vi "FaultCheck.vi"(8 "error in (no error)":errorcluster, 10 "Cluster in":T2, 11 "Enum in":T1) -> (0 "error out":errorcluster, 2 "Cluster out":T2, 3 "Enum out":T1)   [LabVIEW 2018]
uses:
  Type_Def Actuator Controls.ctl
  Type_Def_ControlState.ctl
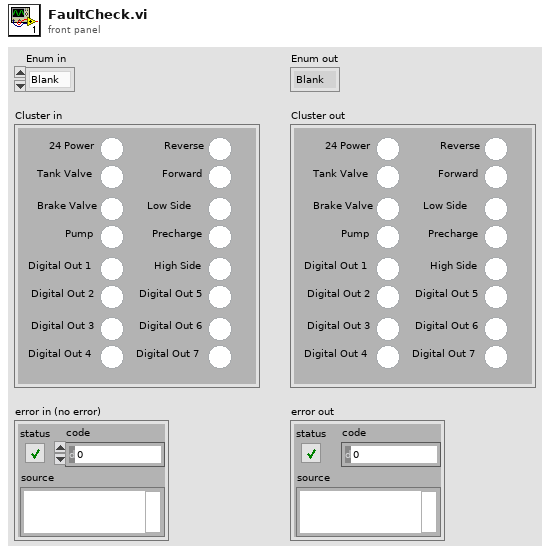
[diagram p1: front panel]
types:
  T1 = typedef "Type_Def_ControlState.ctl" = enum16{"Blank", "Systems Check", "Idle", "Ready", "Pushing", "CrawlingPrecharge", "Braking", "Fault", "Boot Up", "Unpowered", "Crawling", "Shutdown", "Service Push", "Service Wait", "Vent", "Precharge", "Cooldown"}
  T2 = typedef "Type_Def Actuator Controls.ctl" = cluster{"Reverse ":bool, "Forward":bool, "Low Side":bool, "Precharge":bool, "High Side":bool, "Digital Out 5":bool, "Digital Out 6":bool, "Digital Out 7 ":bool, "24 Power":bool, "Tank Valve ":bool, "Brake Valve":bool, "Pump":bool, "Digital Out 1 ":bool, "Digital Out 2":bool, "Digital Out 3":bool, "Digital Out 4 ":bool}
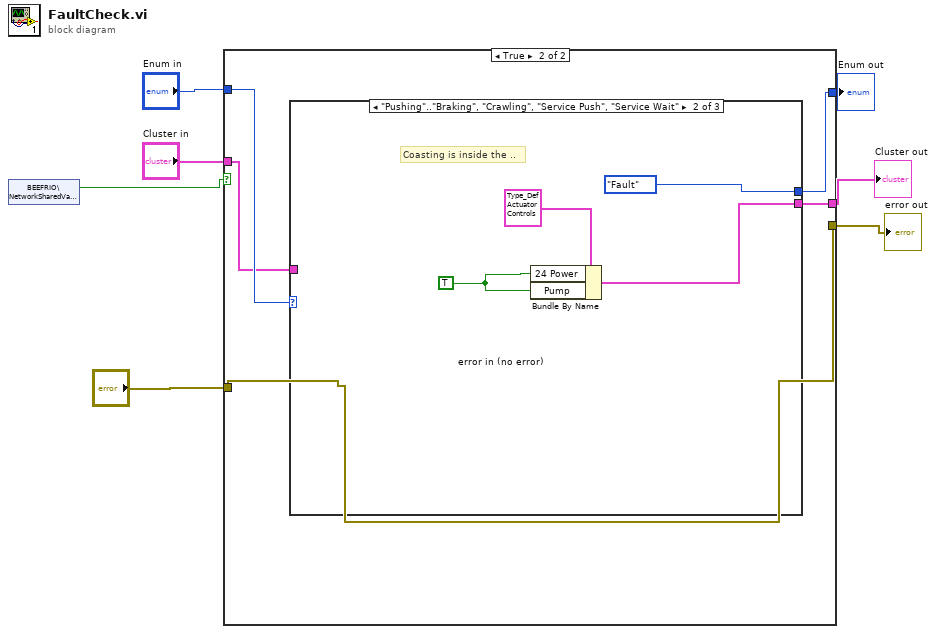
[diagram p0: block diagram]
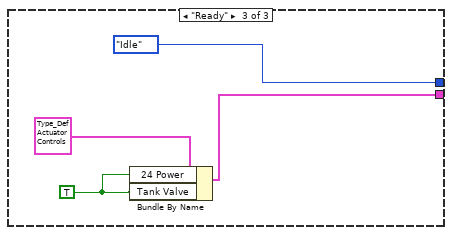
[diagram p4: hidden frame]
diagram:
  n1 = shared-variable "BEEFRIO\\NetworkSharedVariable.lvlib\\Fault"() -> (w1:bool)  [unwired: 1 in, 1 out]
  n2 = case shown="True" w1 {
    tunnel: [w10 w11] -> w7
    tunnel: "error in (no error)" -> [w10 w11]
    tunnel: [w9 w13] -> w5
    tunnel: "Cluster in" -> [w9 w12]
    tunnel: [w8 w14] -> w3
    tunnel: "Enum in" -> [w8 w15]
    frame False {
    }
    frame True {
      n3 = case shown="\"Pushing\"..\"Braking\", \"Crawling\", \"Service Push\", \"Service Wait\"" w15 {
        selector: w15 -> [w16 _ _]
        tunnel: [w16 Type_Def_ControlState."Fault" ("Enum in 2") Type_Def_ControlState."Idle" ("Enum in 2")] -> w14
        tunnel: [w17 w20 w24] -> w13
        tunnel: w12 -> [w17 _ _]
        frame Default {
        }
        frame "Pushing".."Braking", "Crawling", "Service Push", "Service Wait" {
          w18 = TRUE
          # "Coasting is inside the .."
          n4 = Bundle By Name(cluster=T2 {"Reverse "=FALSE, "Forward"=FALSE, "Low Side"=FALSE, "Precharge"=FALSE, "High Side"=FALSE, "Digital Out 5"=FALSE, "Digital Out 6"=FALSE, "Digital Out 7 "=FALSE, "24 Power"=FALSE, "Tank Valve "=FALSE, "Brake Valve"=FALSE, "Pump"=FALSE, "Digital Out 1 "=FALSE, "Digital Out 2"=FALSE, "Digital Out 3"=FALSE, "Digital Out 4 "=FALSE} ("Cluster in 2"), "24 Power"=w18, "Pump"=w18) -> (w20:T2)
        }
        frame "Ready" {
          w22 = TRUE
          n5 = Bundle By Name(cluster=T2 {"Reverse "=FALSE, "Forward"=FALSE, "Low Side"=FALSE, "Precharge"=FALSE, "High Side"=FALSE, "Digital Out 5"=FALSE, "Digital Out 6"=FALSE, "Digital Out 7 "=FALSE, "24 Power"=FALSE, "Tank Valve "=FALSE, "Brake Valve"=FALSE, "Pump"=FALSE, "Digital Out 1 "=FALSE, "Digital Out 2"=FALSE, "Digital Out 3"=FALSE, "Digital Out 4 "=FALSE} ("Cluster in 2"), "24 Power"=w22, "Tank Valve"=w22) -> (w24:T2)
        }
      }
    }
  }
  "error out" <- w7
  "Cluster out" <- w5
  "Enum out" <- w3
